vi "Serial Port Description.vi"(8 "error in (no error)":errorcluster, 11 "Dev Description":string="JLink") -> (0 "error out":errorcluster, 1 "Dev Description":string, 2 "OK?":bool, 3 "VISA resource name":refnum<visa-resource-name>)   [LabVIEW 2018]
uses:
  <vilib>/Instr/_visa.llb/VISA Find Search Mode.ctl
panel:
  out "error in cycle temp":errorcluster
  out "cnt":u8
  out "Devices":string[](array[string])
  out "find list":string[](array[string])
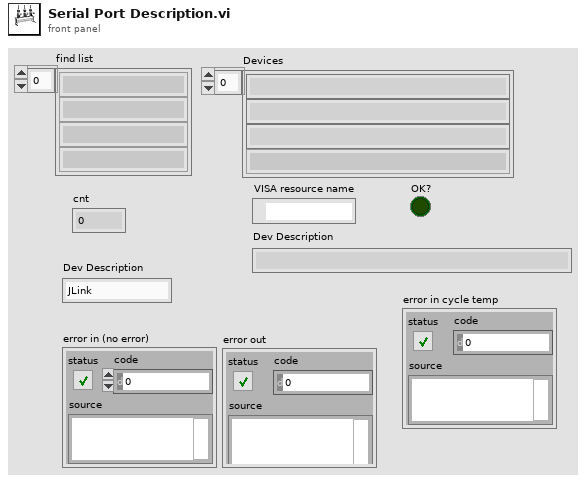
[diagram p1: front panel]
types:
  T1 = typedef "VISA Find Search Mode.ctl" = u32
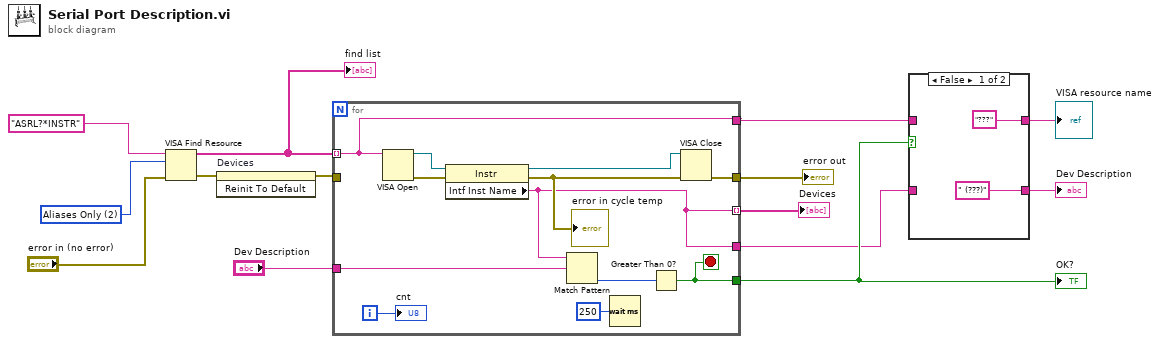
[diagram p0: block diagram]
diagram:
  w14 = T1 2 items=["Canonical Names Only"=0, "Aliases Only"=2, "Include Matching Aliases"=3, "Include All Aliases"=4] ("Search Mode")
  n1 = VISA Find Resource(8:"error in (no error)", 10:w14, 11:"ASRL?*INSTR" ("expression (\"?*\")")) -> (0:w4:errorcluster, 3:w12:string[])  [unwired: 1 out]
  "find list" <- w12
  n2 = invoke on="Devices" class="Arr (strict)" method="Reinit To Default"(error in=w4) -> (error out=w5:errorcluster)  [unwired: 2 in, 2 out]
  n3 = for {
    tunnel: w12 -> [w20] mode=indexing
    tunnel: [w18] -> w11 mode=indexing
    tunnel: [w20] -> w7
    tunnel: [w19] -> w8
    tunnel: [w18] -> w1
    tunnel: w5 -> [_]
    tunnel: [w22] -> w10
    tunnel: "Dev Description" -> [w15]
    i -> [w16]
    stop <- w19 stop-if-true
    n4 = VISA Open(VISA resource name=w20) -> (VISA resource name=w26:refnum<visa-resource-name>, error out=w25:errorcluster)  [unwired: 4 in]
    n5 = property class="Instr"(reference=w26, error in=w25) -> (reference out=w24:refnum<visa-resource-name>, error out=w23:errorcluster, "Intf Inst Name"=w18:string)
    "error in cycle temp" <- w23
    n6 = Match Pattern(string=w18, regular expression=w15) -> (offset past match=w21:i32)  [unwired: 1 in, 3 out]
    n7 = Wait (ms)(milliseconds to wait=u32 250) -> ()  [unwired: 1 out]
    n8 = Greater Than 0?(x=w21) -> (x > 0?=w19:bool)
    n9 = VISA Close(VISA resource name=w24, error in (no error)=w23) -> (error out=w22:errorcluster)
    "cnt" <- w16
  }
  "Devices" <- w11
  "error out" <- w10
  "OK?" <- w8
  n10 = case shown="False" w8 {
    tunnel: w7 -> [_ w30]
    tunnel: ["???" w30] -> w6
    tunnel: [" (???)" w29] -> w2
    tunnel: w1 -> [_ w29]
    frame False {
    }
    frame True {
    }
  }
  "VISA resource name" <- w6
  "Dev Description" <- w2
